vi "flash_RPCV1.vi"() -> ()   [LabVIEW 2017]
panel:
  out "error out 2":errorcluster
  out "Out 2":u8=4 format="%.0x"
  in  "Firmware":u16(ring)=4 items=["SP6"=4, "Middle"=3, "Final"=2]
  out "Out":u8 format="%.0x"
  out "字符串 2":string
  out "concatenated string":string
  in  "Register_Base_Address":u32=512 format="%x"
  in  "start":bool=TRUE
  out "Current IP address":string="192.168.10.20"
  in  "IP address list":string[](array[string])=["192.168.10.20"]
  in  "回读":bool
  out "Current Progress":u32(slide)=342016 scale=0.0..341988.0
  out "error out":errorcluster={"status"=TRUE, "code"=4, "source"="Read from Binary File in flash_RPCV1.vi<APPEND>\nG:\\rpc\\FPGA\\top.bin"}
  out "appended array":bool[](array[boolean])
  out "Process":u32=342016
  in  "error in (no error)":errorcluster
  in  "Read (TRUE)":bool
  out "byte data":string
  out "Total size (in bytes)":i64=341988
  in  "file path (use dialog)":path=path "G:/rpc/FPGA/top_sp6.bin"
  # "FF80 0001 0000 0209 13"
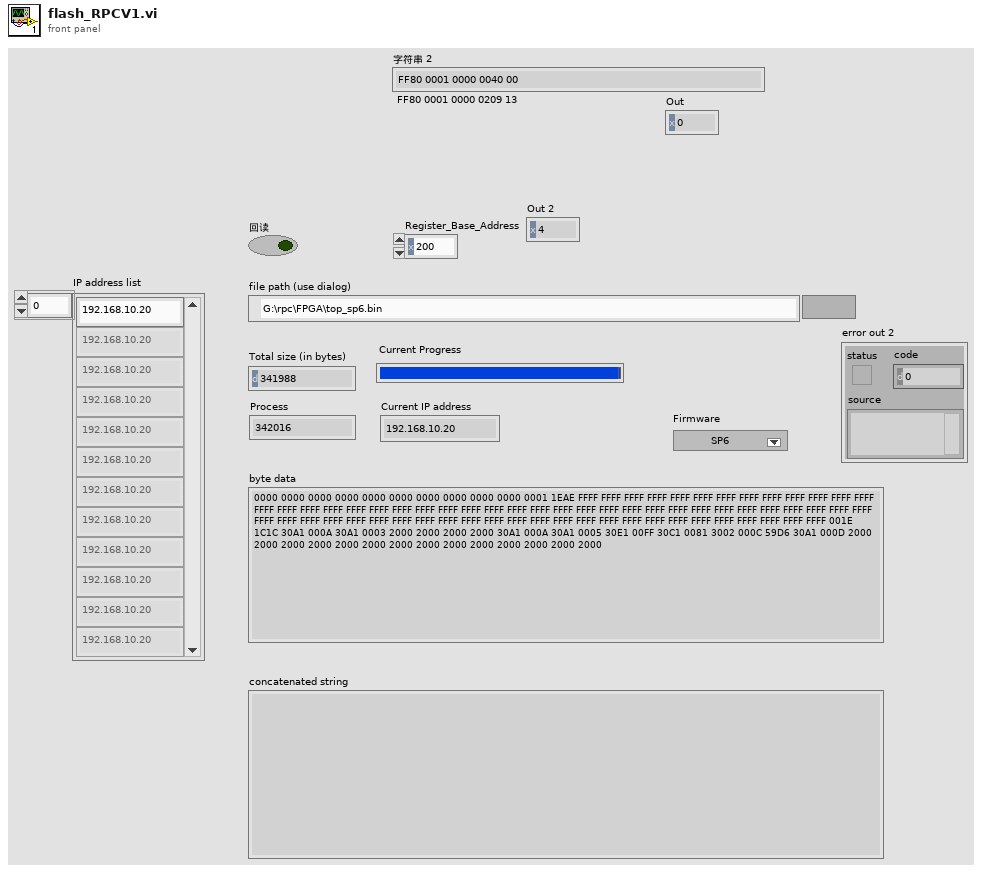
[diagram p1: front panel]
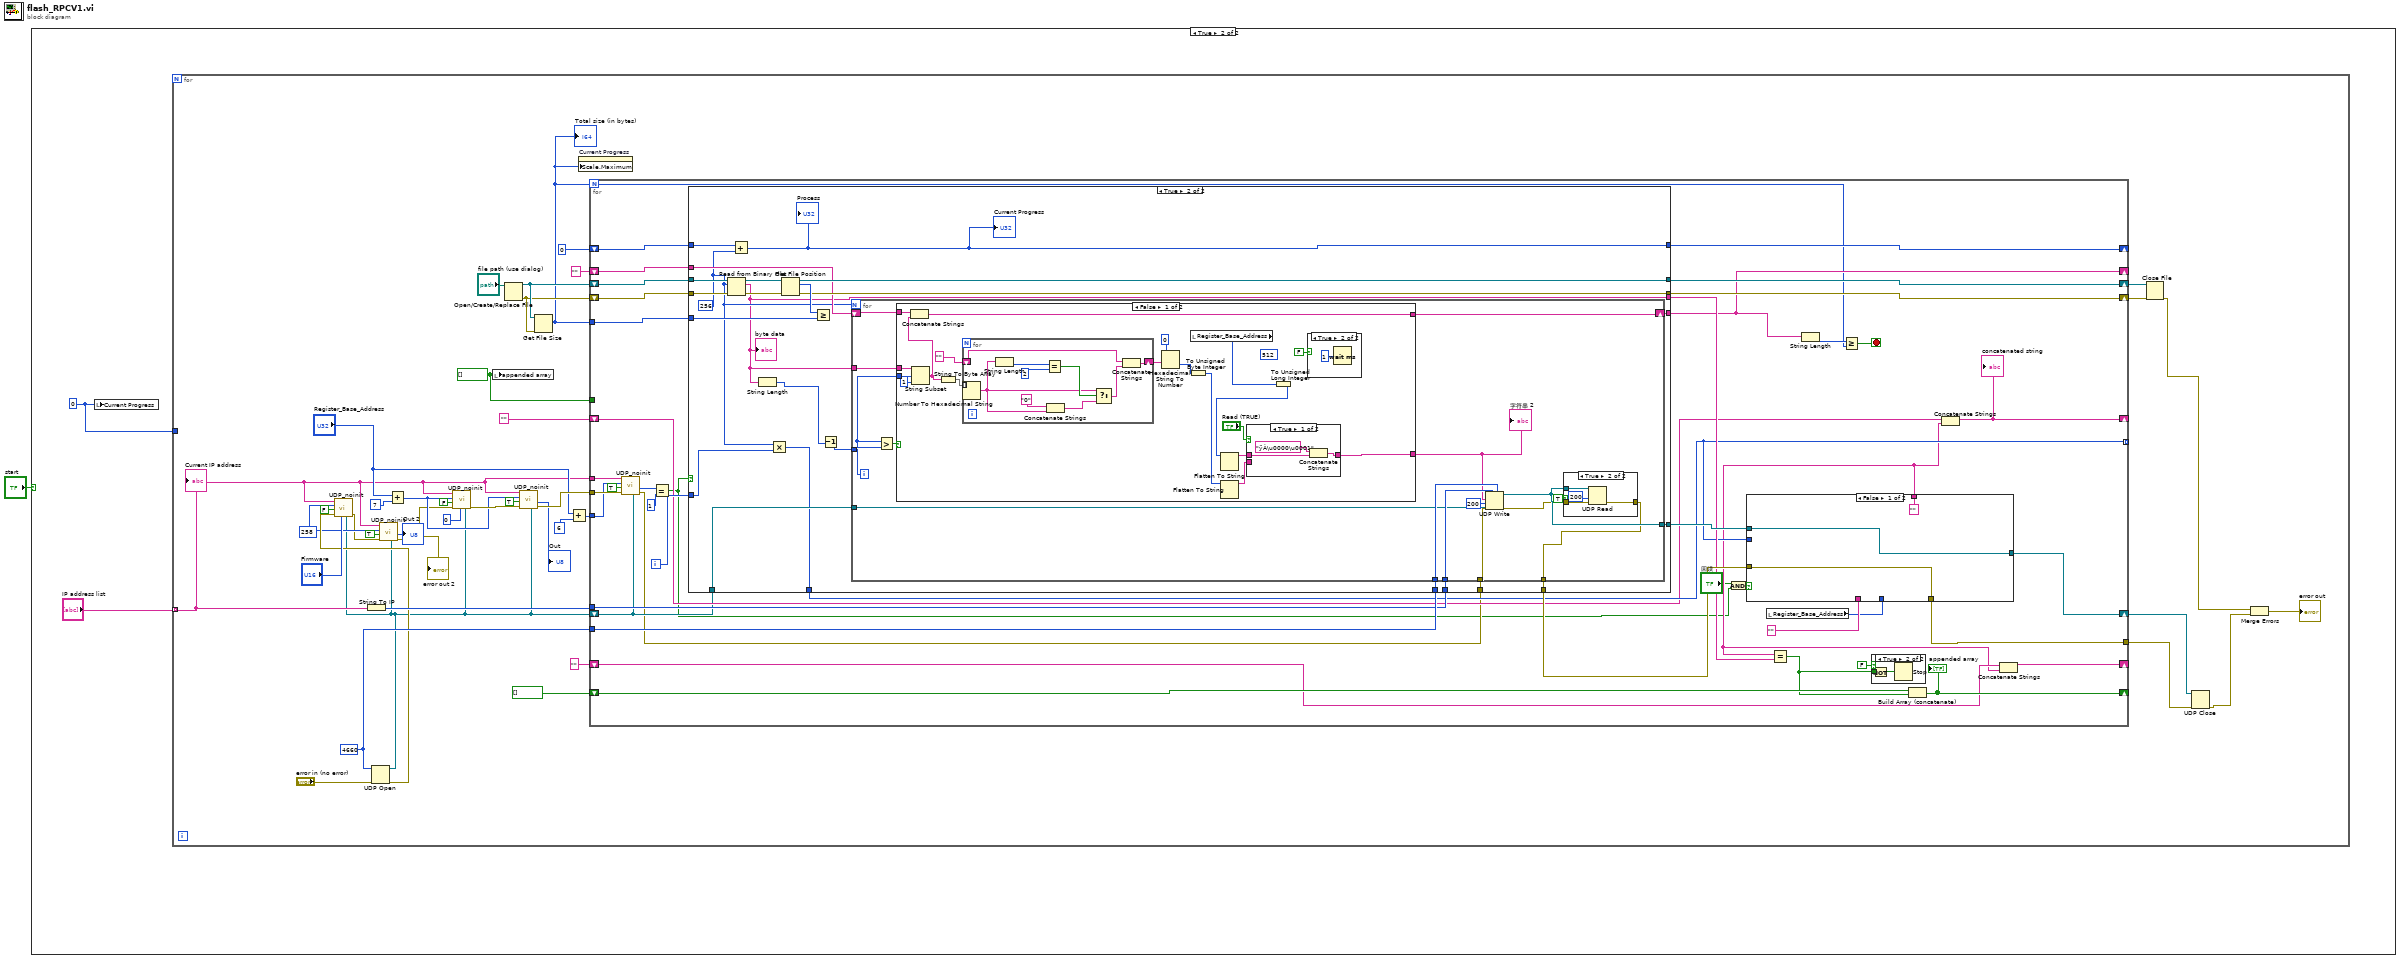
[diagram p0: block diagram]
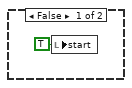
[diagram p2: hidden frame]
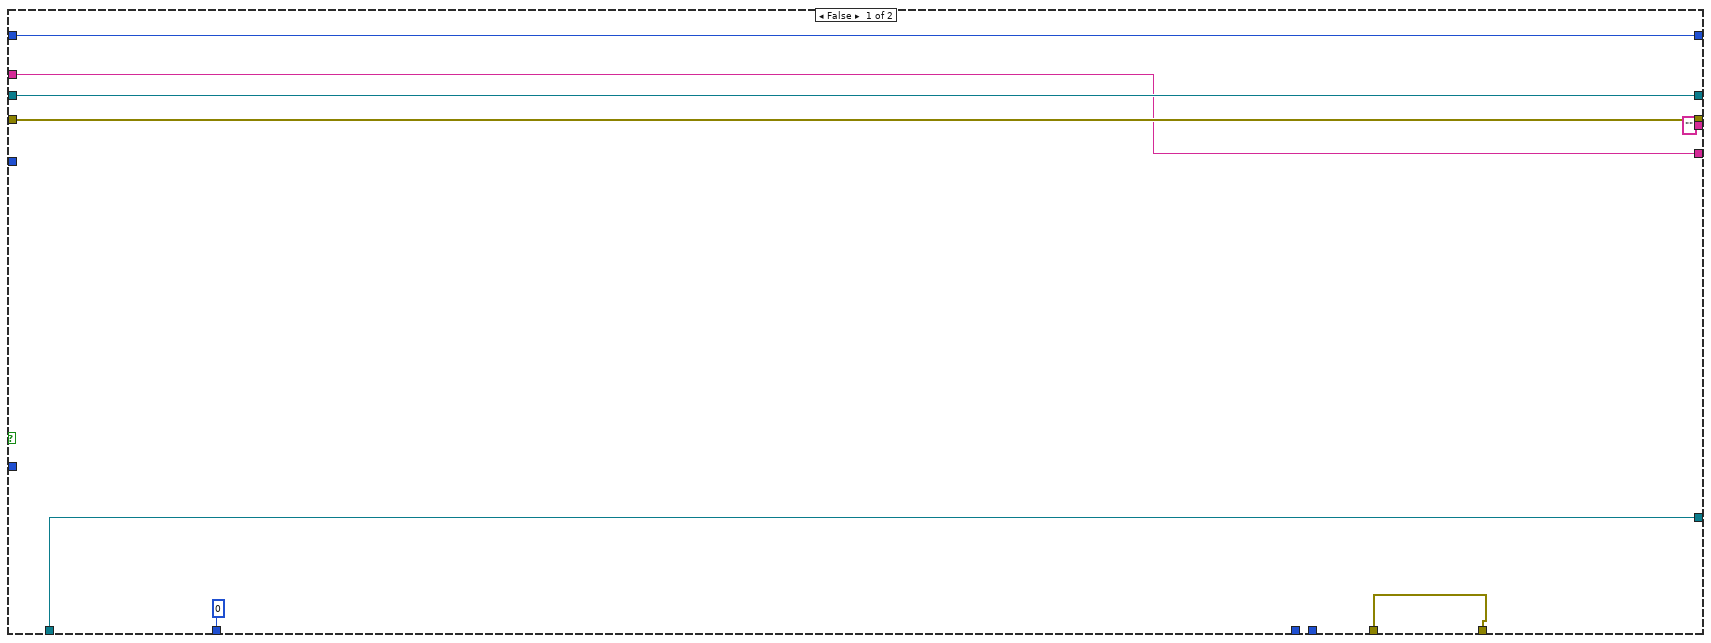
[diagram p3: hidden frame]
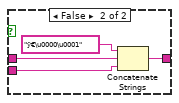
[diagram p5: hidden frame]
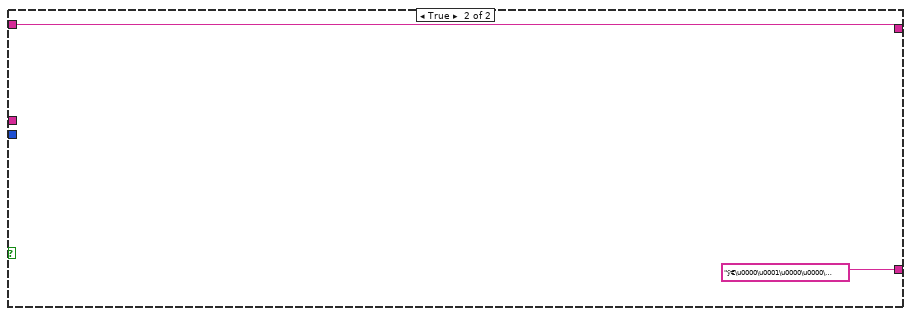
[diagram p7: hidden frame]
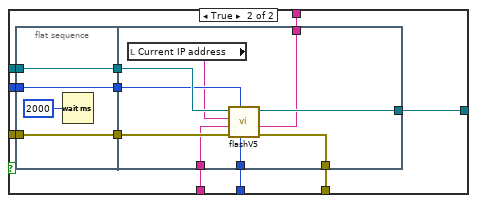
[diagram p8: hidden frame]
diagram:
  n1 = case shown="True" "start" {
    frame False {
      n2 = local write "start"(TRUE ("start")) -> ()
    }
    frame True {
      w3 = u8 0 ("In")
      n3 = local write "Current Progress"(w3) -> ()
      n4 = for {
        tunnel: "IP address list" -> [w11] mode=indexing
        tunnel: w3 -> [_]
        w10 = u32 258 ("Address")
        w25 = bool[] [] ("appended array")
        w40 = u16 4660 ("UDP port")
        n5 = String To IP(1:w11) -> (0:w37:u32)
        n6 = UDP Open(8:"error in (no error)", 11:w40) -> (port=w7:refnum<k16>, 0:w12:errorcluster)  [unwired: 3 in, 1 out]
        n7 = call "UDP_noinit.vi"("connection ID"=w7, "In"="Firmware", "error in (no error)"=w12, "Read (TRUE)"=FALSE, "Address"=w10, "IP address"=w11) -> ("error out"=w6:errorcluster)  [unwired: 2 in, 2 out]
        n8 = call "UDP_noinit.vi"("connection ID"=w7, "error in (no error)"=w6, "Read (TRUE)"=TRUE, "Address"=w10, "IP address"=w11) -> ("error out"=w5:errorcluster, "Out"=→"Out 2":u8)  [unwired: 3 in, 1 out]
        "error out 2" <- w5
        n9 = Add(x="Register_Base_Address", y=u32 7 ("Address")) -> (x+y=w20:u32)
        n10 = call "UDP_noinit.vi"("connection ID"=w7, "In"=u8 0, "error in (no error)"=w5, "Read (TRUE)"=FALSE, "Address"=w20, "IP address"=w11) -> ("error out"=w29:errorcluster)  [unwired: 2 in, 2 out]
        n11 = local write "appended array"(w25) -> ()
        n12 = Open/Create/Replace File(file path (use dialog)="file path (use dialog)") -> (refnum out=w44:refnum<file>, error out=w43:errorcluster)  [unwired: 5 in, 1 out]
        n13 = call "UDP_noinit.vi"("connection ID"=w7, "error in (no error)"=w29, "Read (TRUE)"=TRUE, "Address"=w20, "IP address"=w11) -> ("error out"=w31:errorcluster, "Out"=→"Out":u8)  [unwired: 3 in, 1 out]
        n14 = Get File Size(file=w44, error in=w43) -> (size (in bytes)=w26:i64)  [unwired: 2 out]
        "Total size (in bytes)" <- w26
        n15 = Add(x="Register_Base_Address", y=u32 6 ("Address")) -> (x+y=w17:u32)
        n16 = property on="Current Progress" class="Slide (strict)"("Scale.Maximum"=w26) -> ()  [unwired: 2 in, 2 out]
        n17 = for {
          N: w26 -> [w65]
          tunnel: w26 -> [w86]
          shift-right: [w85] -> w42
          shift-left: w43 -> [w87]
          shift-right: [w84] -> w41
          shift-left: w44 -> [w88]
          shift-right: [w67] -> _
          shift-left: "" -> [w83]
          tunnel: w40 -> [w80]
          tunnel: [w75] -> w38
          tunnel: w37 -> [w79]
          shift-right: [w77] -> w39
          shift-left: w7 -> [w55]
          shift-right: [w81] -> _
          shift-left: u32 0 ("length (rest)") -> [w82]
          shift-right: [w72] -> _
          shift-left: bool[] [] -> [w70]
          tunnel: [w68] -> _ mode=indexing
          shift-right: [w63] -> _
          shift-left: "" -> [w62]
          tunnel: w11 -> [w60]
          tunnel: w31 -> [w54]
          shift-right: [w52] -> _
          shift-left: "" -> [w51]
          tunnel: w25 -> [_]
          tunnel: w17 -> [w47]
          i -> [w73]
          stop <- w64 stop-if-true
          n18 = call "UDP_noinit.vi"("connection ID"=w55, "error in (no error)"=w54, "Read (TRUE)"=TRUE, "Address"=w47, "IP address"=w60) -> ("error out"=w53:errorcluster, "Out"=w58:u8)  [unwired: 3 in, 1 out]
          n19 = Equal?(x=w58, y=u8 1) -> (x = y?=w49:bool)
          n20 = case shown="True" w49 {
            tunnel: w88 -> [w93 w120]
            tunnel: w87 -> [w94 w119]
            tunnel: w86 -> [_ w115]
            tunnel: [w94 w114] -> w85
            tunnel: [w93 w113] -> w84
            tunnel: w83 -> [w91 w112]
            tunnel: w82 -> [w92 w111]
            tunnel: [w92 w97] -> w81
            tunnel: w80 -> [_ w110]
            tunnel: w79 -> [_ w109]
            tunnel: w53 -> [w95 w108]
            tunnel: w55 -> [w96 w107]
            tunnel: [w96 w104] -> w78
            tunnel: [w95 w103] -> w76
            tunnel: w73 -> [_ w102]
            tunnel: ["" w100] -> w71
            tunnel: [0 w99] -> w68
            tunnel: [w91 w98] -> w67
            frame False {
            }
            frame True {
              w101 = 256 ("count (1)")
              n21 = Read from Binary File(8:w119, 10:w101, 11:w120) -> (0:w117:errorcluster, 2:w100:string, 3:w118:refnum<file>)  [unwired: 3 in, 1 out]
              "byte data" <- w100
              n22 = Add(x=w111, y=w101) -> (x+y=w97:u32)
              "Process" <- w97
              "Current Progress" <- w97
              n23 = String Length(string=w100) -> (length=w106:i32)
              n24 = Multiply(x=w101, y=w102) -> (x*y=w99:i32)
              n25 = Get File Position(4:w117, 7:w118) -> (0:w114:errorcluster, 2:w116:i64, 3:w113:refnum<file>)
              n26 = Greater Or Equal?(x=w116, y=w115) -> ()  [unwired: 1 out]
              n27 = Decrement(x=w106) -> (x-1=w105:i32)
              n28 = for {
                N: w101 -> [_]
                tunnel: w100 -> [w136]
                shift-right: [w134] -> w98
                shift-left: w112 -> [w135]
                tunnel: w110 -> [w133]
                tunnel: w109 -> [w132]
                tunnel: w108 -> [w131]
                tunnel: w107 -> [w125]
                tunnel: [w121] -> w103
                tunnel: [w124] -> w104
                tunnel: w105 -> [w128]
                i -> [w127]
                n29 = Greater?(x=w127, y=w128) -> (0:w129:bool)
                n30 = case shown="False" w129 {
                  tunnel: w136 -> [w153 _]
                  tunnel: w135 -> [w151 w179]
                  tunnel: [w150 w179] -> w134
                  tunnel: w127 -> [w144 _]
                  tunnel: [w143 "ÿ€\u0000\u0001\u0000\u0000\u0000@\u0000" ("字符串 2")] -> w126
                  frame False {
                    (unwired) u32 512 ("Address")
                    n31 = String Subset(string=w153, offset (0)=w144, length (rest)=1 ("length (rest)")) -> (substring=w149:string)
                    n32 = Concatenate Strings(w151, w149) -> (w150:string)
                    n33 = String To Byte Array(string=w149) -> (unsigned byte array=w159:u8[])
                    n34 = for {
                      shift-right: [w177] -> w158
                      shift-left: "" ("format string") -> [w174]
                      tunnel: w159 -> [w178] mode=indexing
                      n35 = Number To Hexadecimal String(2:w178) -> (0:w170:string)  [unwired: 1 in]
                      n36 = String Length(string=w170) -> (length=w176:i32)
                      n37 = Equal?(x=w176, y=2) -> (x = y?=w173:bool)
                      n38 = Concatenate Strings("0" ("format string"), w170) -> (w172:string)
                      n39 = Select(t=w170, s=w173, f=w172) -> (s? t:f=w169:string)
                      n40 = Concatenate Strings(w174, w169) -> (w177:string)
                    }
                    n41 = Hexadecimal String To Number(string=w158, default (0uL)=u64 0 ("default (0 U32)")) -> (number=w156:u64)  [unwired: 1 in, 1 out]
                    n42 = To Unsigned Byte Integer(number=w156) -> (unsigned 8bit integer=w155:u8)
                    n43 = local read "Register_Base_Address"() -> (w142:u32)
                    n44 = Flatten To String(anything=w155) -> (data string=w146:string)  [unwired: 3 in, 2 out]
                    n45 = To Unsigned Long Integer(number=w142) -> (unsigned 32bit integer=w154:u32)
                    n46 = Flatten To String(anything=w154) -> (data string=w147:string)  [unwired: 3 in, 2 out]
                    n47 = case shown="True" "Read (TRUE)" {
                      tunnel: [w162 w166] -> w143
                      tunnel: w147 -> [w161 w165]
                      tunnel: w146 -> [_ w164]
                      frame True {
                        n48 = Concatenate Strings("ÿÀ\u0000\u0001" ("initial string"), w161) -> (w162:string)
                      }
                      frame False {
                        n49 = Concatenate Strings("ÿ€\u0000\u0001" ("initial string"), w165, w164) -> (w166:string)
                      }
                    }
                    n50 = case shown="True" FALSE {
                      frame False {
                      }
                      frame True {
                        n51 = Wait (ms)(milliseconds to wait=u32 1) -> ()  [unwired: 1 out]
                      }
                    }
                  }
                  frame True {
                  }
                }
                "字符串 2" <- w126
                n52 = UDP Write(address=w132, port or service name=w133, connection ID=w125, data in=w126, 8:w131, 9:200 ("timeout ms (25000)")) -> (error out=w122:errorcluster, 3:w124:refnum<k16>)
                n53 = case shown="True" TRUE {
                  tunnel: w124 -> [_ w141]
                  tunnel: w122 -> [w137 w140]
                  tunnel: [w137 w139] -> w121
                  frame False {
                  }
                  frame True {
                    n54 = UDP Read(connection ID=w141, timeout ms (25000)=200, 8:w140) -> (error out=w139:errorcluster)  [unwired: 5 out]
                  }
                }
              }
            }
          }
          n55 = And(x="回读", y=w49) -> (x .and. y?=w56:bool)
          n56 = local read "Register_Base_Address"() -> (w46:u32)
          n57 = case shown="False" w56 {
            tunnel: w78 -> [w183 w191]
            tunnel: [w183 w190] -> w77
            tunnel: w76 -> [w182 w189]
            tunnel: [w182 w188] -> w75
            tunnel: "" ("empty") -> [_ w187]
            tunnel: w68 -> [_ w186]
            tunnel: ["" ("String") w185] -> w50
            tunnel: w46 -> [_ w184]
            frame False {
            }
            frame True {
              n58 = flat-sequence {
                tunnel: w186 -> [w196]
                tunnel: w189 -> [w197]
                tunnel: w191 -> [w198]
                tunnel: [w198] -> w194
                tunnel: [w197] -> w193
                tunnel: [w196] -> w192
                tunnel: [w204] -> w188
                tunnel: w187 -> [w203]
                tunnel: [w202] -> w185
                tunnel: w194 -> [w207]
                tunnel: w193 -> [w205]
                tunnel: w192 -> [w201]
                tunnel: [w206] -> w190
                tunnel: w184 -> [w199]
                frame #0 {
                  n59 = Wait (ms)(milliseconds to wait=u32 2000) -> ()  [unwired: 1 out]
                }
                frame #1 {
                  n60 = local read "Current IP address"() -> (w200:string)
                  n61 = call "flashV5.vi"("Register_Base_Address"=w199, "flash_base_address"=w201, "error in (no error)"=w205, "empty"=w203, "address"=w200, "connection ID"=w207) -> ("error out"=w204:errorcluster, "String"=w202:string, "connection ID 2"=w206:refnum<k16>)  [unwired: 2 in, 1 out]
                }
              }
            }
          }
          n62 = Equal?(x=w50, y=w71) -> (x = y?=w69:bool)
          n63 = String Length(string=w67) -> (length=w66:i32)
          n64 = Greater Or Equal?(x=w66, y=w65) -> (x >= y?=w64:bool)
          n65 = case shown="True" FALSE {
            tunnel: w69 -> [_ w208]
            frame False {
            }
            frame True {
              n66 = Not(x=w208) -> (.not. x?=w209:bool)
              n67 = Stop(stop? (T)=w209) -> ()
            }
          }
          n68 = Build Array (concatenate)(w70, w69) -> (w72:bool[])
          "appended array" <- w72
          n69 = Concatenate Strings(w62, w50) -> (w63:string)
          "concatenated string" <- w63
          n70 = Concatenate Strings(w51, w50) -> (w52:string)
        }
        n71 = Close File(refnum=w41, error in=w42) -> (error out=w24:errorcluster)  [unwired: 1 out]
        n72 = UDP Close(connection ID=w39, 8:w38) -> (error out=w23:errorcluster)  [unwired: 1 out]
        n73 = Merge Errors(w24, w23) -> (→"error out":errorcluster)
        "Current IP address" <- w11
      }
    }
  }
